vi "Software Update HCC Get Board IDs and Locations.vi"(7 "Debug":bool, 8 "Error In":errorcluster, 11 "Newfi Exe Folder Path":path) -> (0 "Error Out":errorcluster, 1 "Board Index":i32[](array[numeric]), 3 "Active Stations with Board IDs":string[][](array[string]), 4 "All Station Labels":string[](array[string]))   [LabVIEW 2016]
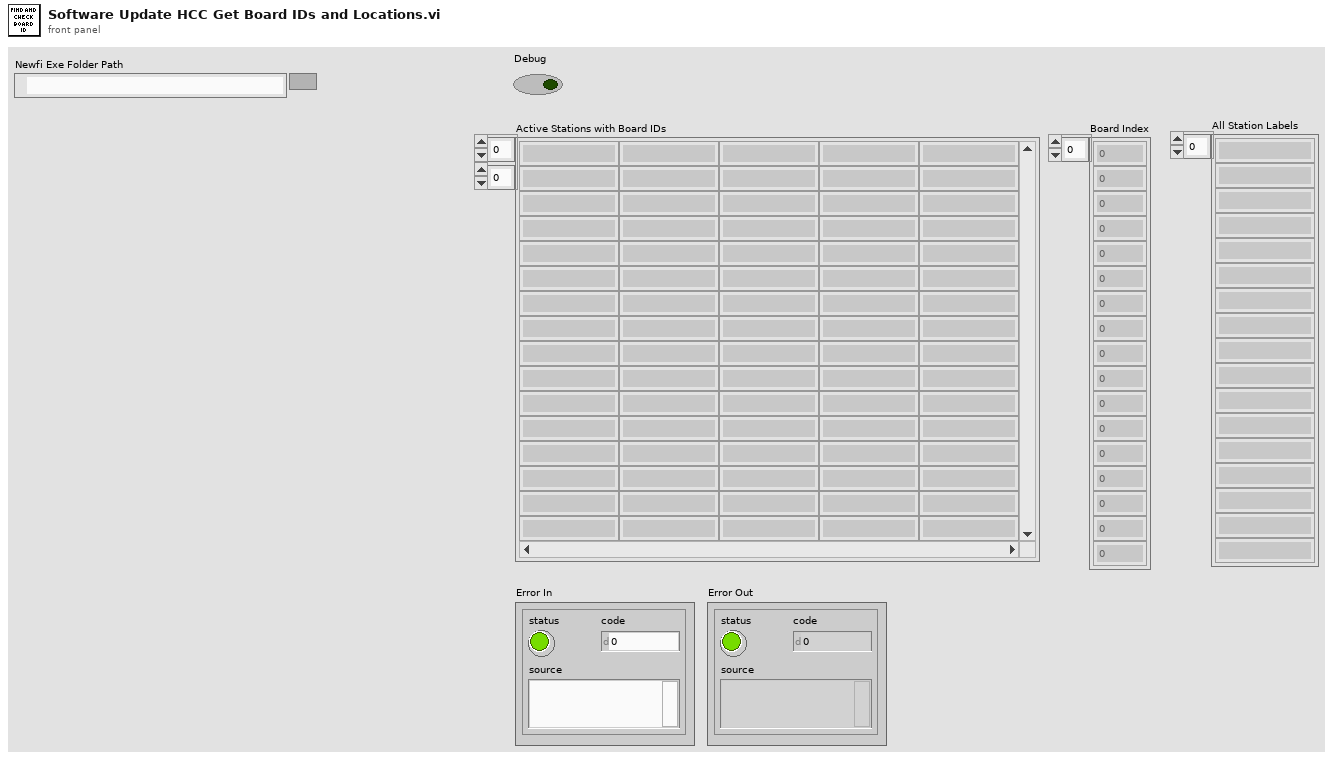
[diagram p1: front panel]
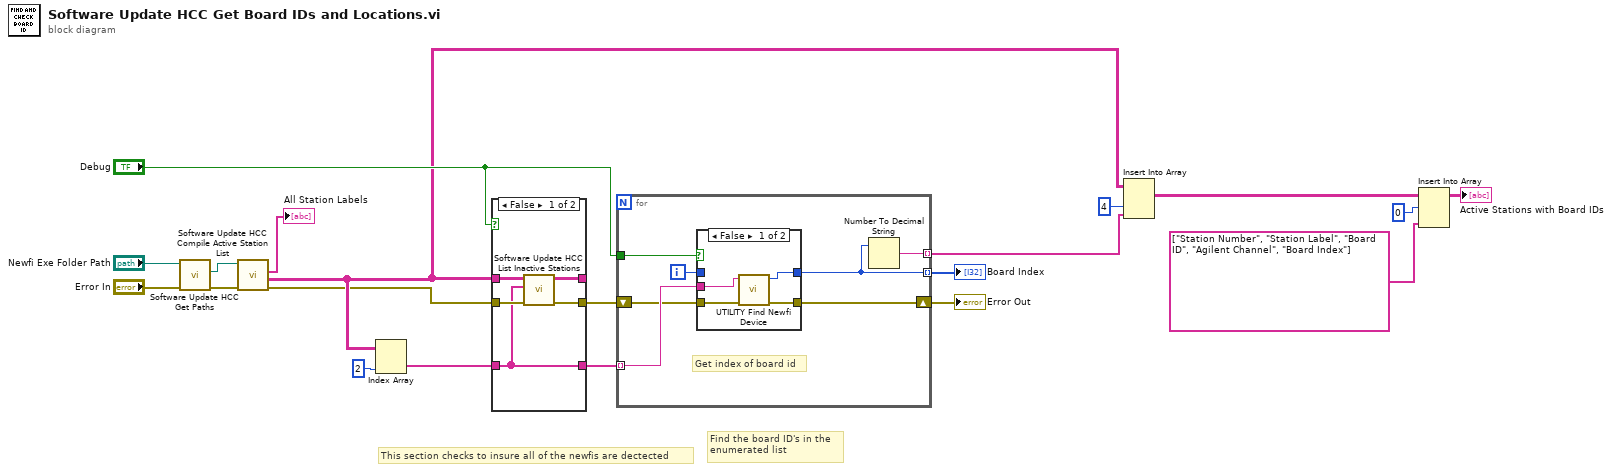
[diagram p0: block diagram]
diagram:
  # "Find the board ID's in the\nenumerated list"
  # "This section checks to insure all of the newfis are dectected"
  n1 = call "Software Update HCC Get Paths.vi"("Error In"="Error In", "Newfi Exe Folder Path"="Newfi Exe Folder Path") -> ("Error Out"=w3:errorcluster, "Stations and Board IDs"=w4:path)  [unwired: 7 in, 1 out]
  n2 = call "Software Update HCC Compile Active Station List.vi"("Error In"=w3, "Station And Board ID Path"=w4) -> ("Error Out"=w1:errorcluster, "List of Stations"=w16:string[][], "All Station Labels"=→"All Station Labels":string[])  [unwired: 7 in]
  n3 = Index Array(array=w16, index (col)=2 ("disabled index (col)")) -> (element=w15:string[])  [unwired: 1 in]
  n4 = case shown="False" "Debug" {
    tunnel: w1 -> [w25 w28]
    tunnel: [w24 w28] -> w20
    tunnel: [w21 w27] -> w19
    tunnel: [w23 w26] -> _
    tunnel: w16 -> [w22 w26]
    tunnel: w15 -> [w21 w27]
    frame False {
      n5 = call "Software Update HCC List Inactive Stations.vi"("error in (no error)"=w25, "List of Stations"=w21, "List of Stations 2"=w22) -> ("error out"=w24:errorcluster, "Array"=w23:string[][])  [unwired: 7 in]
    }
    frame True {
    }
  }
  n6 = for {
    tunnel: w19 -> [w35] mode=indexing
    shift-right: [w33] -> w13
    shift-left: w20 -> [w34]
    tunnel: [w32] -> w12 mode=indexing
    tunnel: "Debug" -> [w31]
    tunnel: [w29] -> w6 mode=indexing
    i -> [w30]
    # "Get index of board id"
    n7 = case shown="False" w31 {
      tunnel: w35 -> [w39 _]
      tunnel: w34 -> [w38 w40]
      tunnel: [w37 w40] -> w33
      tunnel: [w36 w41] -> w29
      tunnel: w30 -> [_ w41]
      frame False {
        n8 = call "UTILITY Find Newfi Device.vi"("error in (no error)"=w38, "Board ID Config"=w39) -> ("error out"=w37:errorcluster, "Current Board Index"=w36:i32)  [unwired: 6 in, 2 out]
      }
      frame True {
      }
    }
    n9 = Number To Decimal String(number=w29) -> (decimal integer string=w32:string)  [unwired: 1 in]
  }
  "Error Out" <- w13
  "Board Index" <- w6
  n10 = Insert Into Array(array=w16, index (col)=4 ("disabled index (col)"), new element=w12) -> (w10:string[][])  [unwired: 1 in]
  n11 = Insert Into Array(array=w10, index (row)=0, new element=string[] ["Station Number", "Station Label", "Board ID", "Agilent Channel", "Board Index"]) -> (→"Active Stations with Board IDs":string[][])  [unwired: 1 in]
